vi "Init_references.vi"(8 "error in":errorcluster, 11 "Application":refnum<k7>) -> (0 "error out":errorcluster, 3 "References":T1)   [LabVIEW 2016]
uses:
  References.ctl
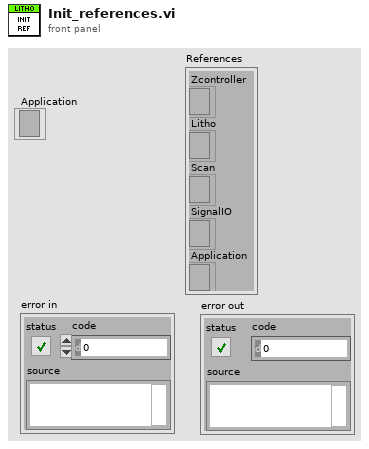
[diagram p1: front panel]
types:
  T1 = typedef "References.ctl" = cluster{"Zcontroller":refnum<k7>, "Litho":refnum<k7>, "Scan":refnum<k7>, "SignalIO":refnum<k7>, "Application":refnum<k7>}
  T2 = cluster{"Zcontroller":refnum<k7>, "Litho":refnum<k7>, "Scan":refnum<k7>, "SignalIO":refnum<k7>, "Application":refnum<k7>}
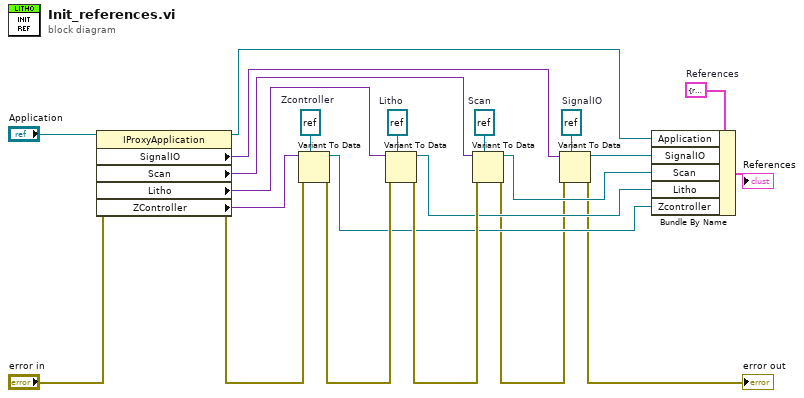
[diagram p0: block diagram]
diagram:
  w5 = T2 {"Zcontroller"=refnum, "Litho"=refnum, "Scan"=refnum, "SignalIO"=refnum, "Application"=refnum}  # References
  w19 = refnum<k7> refnum  # SignalIO
  w20 = refnum<k7> refnum  # Scan
  w21 = refnum<k7> refnum  # Litho
  w22 = refnum<k7> refnum  # Zcontroller
  n1 = property class="IProxyApplication"(reference="Application", error in="error in") -> (reference out=w1:refnum<k7>, error out=w18:errorcluster, "SignalIO"=w17:variant, "Scan"=w16:variant, "Litho"=w15:variant, "ZController"=w14:variant)
  n2 = Variant To Data(error in=w18, type=w22, Variant=w14) -> (data=w10:refnum<k7>, error out=w13:errorcluster)
  n3 = Variant To Data(error in=w13, type=w21, Variant=w15) -> (data=w9:refnum<k7>, error out=w12:errorcluster)
  n4 = Variant To Data(error in=w12, type=w20, Variant=w16) -> (data=w8:refnum<k7>, error out=w7:errorcluster)
  n5 = Variant To Data(error in=w7, type=w19, Variant=w17) -> (data=w11:refnum<k7>, error out=→"error out":errorcluster)
  n6 = Bundle By Name(cluster=w5, "Application"=w1, "SignalIO"=w11, "Scan"=w8, "Litho"=w9, "Zcontroller"=w10) -> (→"References":T2)
